vi "validate_controls.vi"(8 "error in (no error)":errorcluster, 11 "ScanModeTS090821Circular2D in":refnum<class "ImagingModeTS090821Circular2D.lvclass">) -> (0 "error out":errorcluster, 3 "ScanModeTS090821Circular2D out":refnum<class "ImagingModeTS090821Circular2D.lvclass">)   [LabVIEW 2010, in "ImagingModeTS090821Circular2D.lvclass"]
uses:
  ImagingModeTS090821Circular2D.lvclass
  ImagingModeTS090821Circular2D.lvclass/ImagingModeTS090821Circular2D.ctl
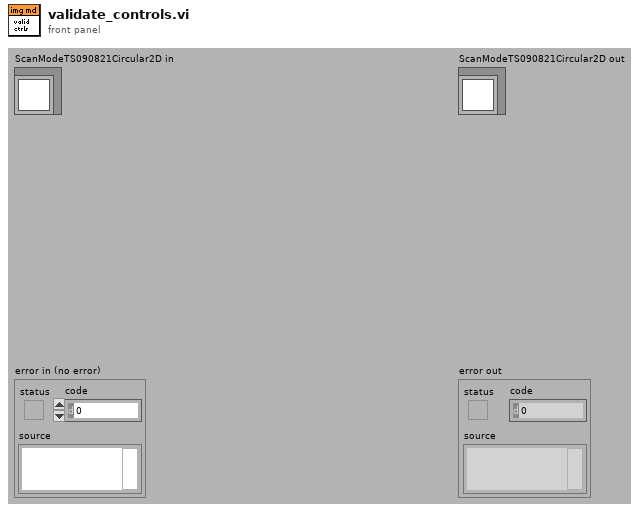
[diagram p1: front panel]
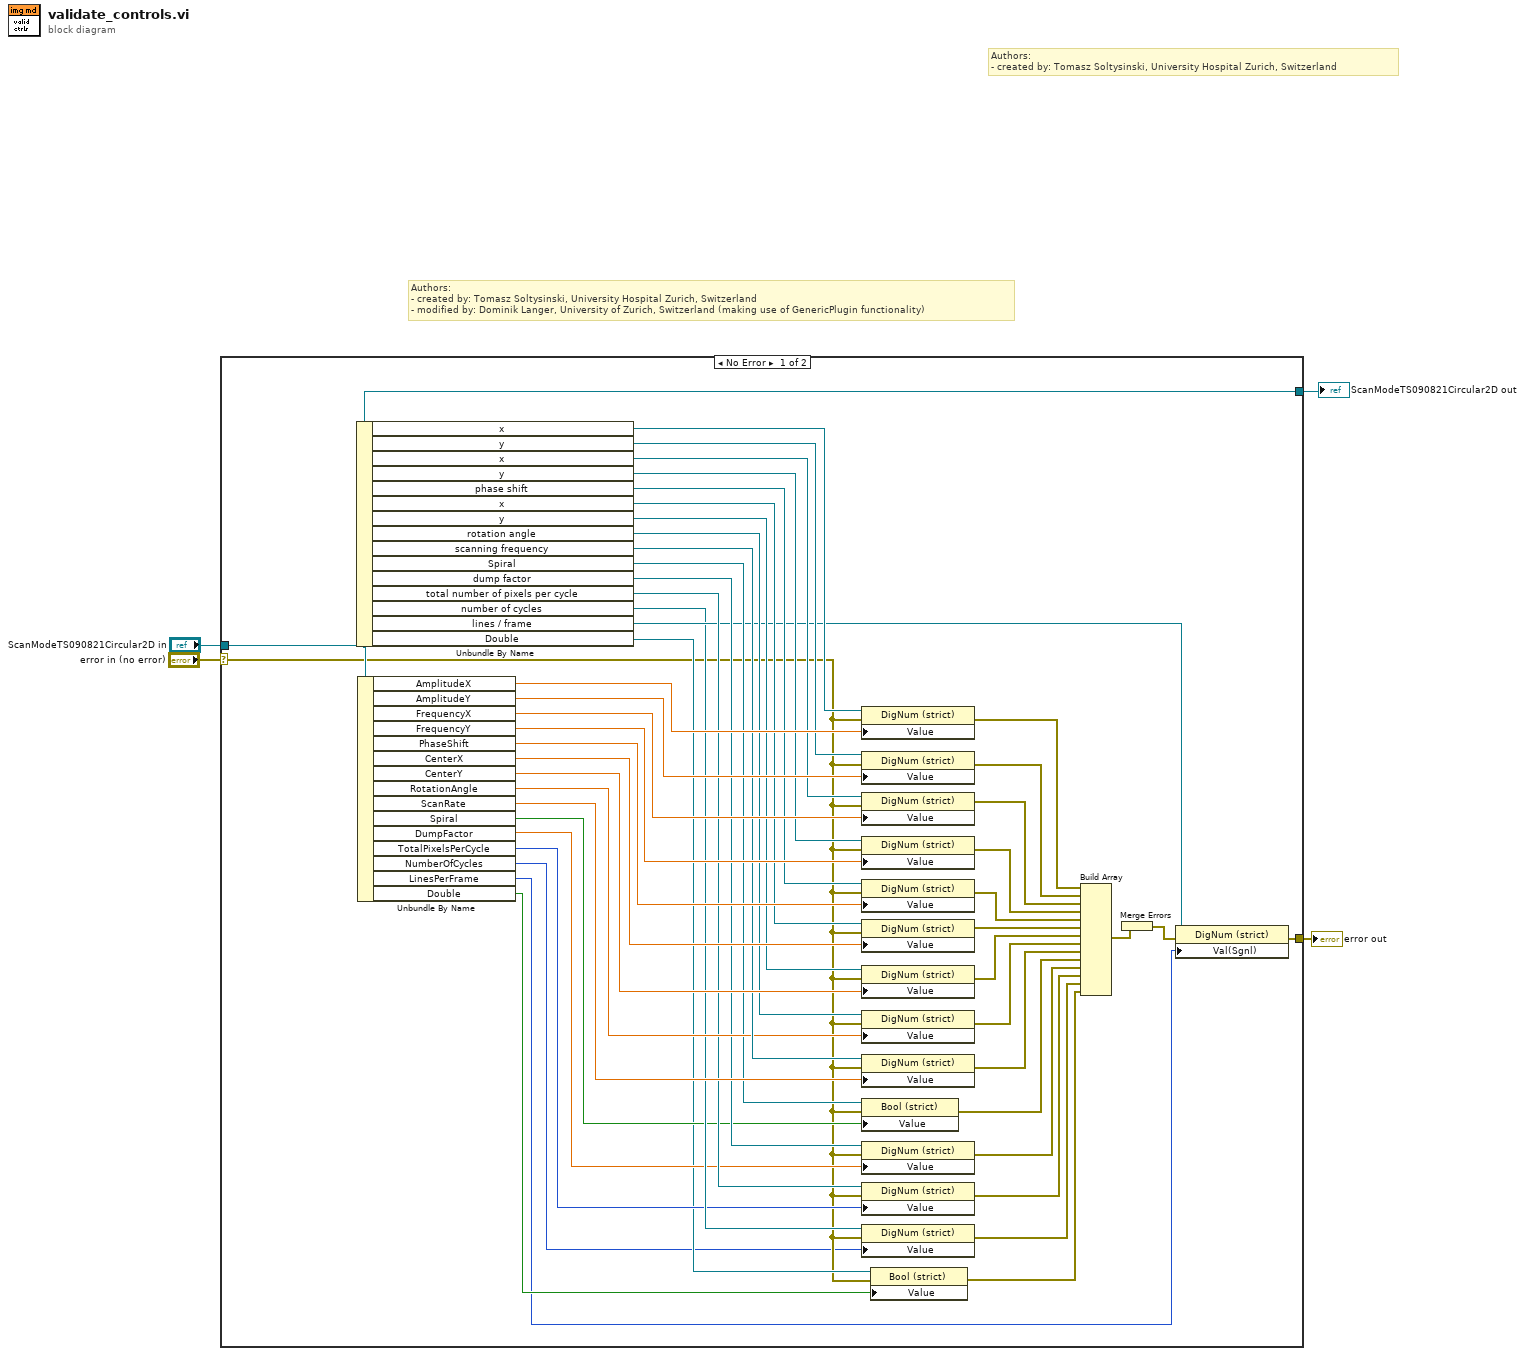
[diagram p0: block diagram]
diagram:
  # "Authors: \n- created by: Tomasz Soltysinski, University Hospital Zurich, Switzerland\n- modified by: Dominik Langer, University of Zurich, Switzerland (making use of GenericPlugin functionality)"
  # "Authors: \n- created by: Tomasz Soltysinski, University Hospital Zurich, Switzerland"
  n1 = case shown="No Error" "error in (no error)" {
    selector: "error in (no error)" -> [w8 w55]
    tunnel: [w51 w55] -> w2
    tunnel: [w12 w54] -> w1
    tunnel: "ScanModeTS090821Circular2D in" -> [w12 w54]
    frame No Error {
      n2 = Unbundle By Name(w12) -> ("x"=w31:refnum<vi>, "y"=w30:refnum<vi>, "x"=w29:refnum<vi>, "y"=w28:refnum<vi>, "phase shift"=w27:refnum<vi>, "x"=w26:refnum<vi>, "y"=w25:refnum<vi>, "rotation angle"=w24:refnum<vi>, "scanning frequency"=w23:refnum<vi>, "Spiral"=w20:refnum<vi>, "dump factor"=w19:refnum<vi>, "total number of pixels per cycle"=w18:refnum<vi>, "number of cycles"=w16:refnum<vi>, "lines / frame"=w17:refnum<vi>, "Double"=w10:refnum<vi>)
      n3 = Unbundle By Name(w12) -> ("AmplitudeX"=w38:dbl[unit], "AmplitudeY"=w37:dbl[unit], "FrequencyX"=w36:dbl, "FrequencyY"=w35:dbl, "PhaseShift"=w34:dbl, "CenterX"=w33:dbl, "CenterY"=w32:dbl, "RotationAngle"=w22:dbl, "ScanRate"=w21:dbl[unit], "Spiral"=w11:bool, "DumpFactor"=w13:dbl, "TotalPixelsPerCycle"=w14:i32, "NumberOfCycles"=w6:i32, "LinesPerFrame"=w5:i32, "Double"=w9:bool)
      n4 = property class="DigNum (strict)"(reference=w31, error in=w8, "Value"=w38) -> (error out=w50:errorcluster)  [unwired: 1 out]
      n5 = property class="DigNum (strict)"(reference=w30, error in=w8, "Value"=w37) -> (error out=w49:errorcluster)  [unwired: 1 out]
      n6 = property class="DigNum (strict)"(reference=w29, error in=w8, "Value"=w36) -> (error out=w39:errorcluster)  [unwired: 1 out]
      n7 = property class="DigNum (strict)"(reference=w28, error in=w8, "Value"=w35) -> (error out=w48:errorcluster)  [unwired: 1 out]
      n8 = property class="DigNum (strict)"(reference=w27, error in=w8, "Value"=w34) -> (error out=w47:errorcluster)  [unwired: 1 out]
      n9 = property class="DigNum (strict)"(reference=w26, error in=w8, "Value"=w33) -> (error out=w46:errorcluster)  [unwired: 1 out]
      n10 = property class="DigNum (strict)"(reference=w25, error in=w8, "Value"=w32) -> (error out=w45:errorcluster)  [unwired: 1 out]
      n11 = property class="DigNum (strict)"(reference=w24, error in=w8, "Value"=w22) -> (error out=w44:errorcluster)  [unwired: 1 out]
      n12 = property class="DigNum (strict)"(reference=w23, error in=w8, "Value"=w21) -> (error out=w43:errorcluster)  [unwired: 1 out]
      n13 = property class="Bool (strict)"(reference=w20, error in=w8, "Value"=w11) -> (error out=w42:errorcluster)  [unwired: 1 out]
      n14 = property class="DigNum (strict)"(reference=w19, error in=w8, "Value"=w13) -> (error out=w41:errorcluster)  [unwired: 1 out]
      n15 = property class="DigNum (strict)"(reference=w18, error in=w8, "Value"=w14) -> (error out=w40:errorcluster)  [unwired: 1 out]
      n16 = property class="DigNum (strict)"(reference=w16, error in=w8, "Value"=w6) -> (error out=w15:errorcluster)  [unwired: 1 out]
      n17 = property class="Bool (strict)"(reference=w10, error in=w8, "Value"=w9) -> (error out=w7:errorcluster)  [unwired: 1 out]
      n18 = Build Array(w50, w49, w39, w48, w47, w46, w45, w44, w43, w42, w41, w40, w15, w7) -> (w53:errorcluster[])
      n19 = Merge Errors(w53) -> (w52:errorcluster)
      n20 = property class="DigNum (strict)"(reference=w17, error in=w52, "Val(Sgnl)"=w5) -> (error out=w51:errorcluster)  [unwired: 1 out]
    }
    frame Error {
    }
  }
  "error out" <- w2
  "ScanModeTS090821Circular2D out" <- w1
